vi "DeQ Valve State.vi"(8 "error in (no error)":errorcluster, 11 "Capillary Line in":refnum<class "Capillary Line.lvclass">) -> (0 "error out":errorcluster, 3 "Capillary Line out":refnum<class "Capillary Line.lvclass">)   [LabVIEW 2015, in "cRIO-Carbondioxide.lvlib" / "CO2-Actor.lvlib" / "Capillary Line.lvclass"]
uses:
  Capillary Line.lvclass
  Capillary Line.lvclass/Capillary Line.ctl
panel:
  out "timed out?":bool
  out "State":u16
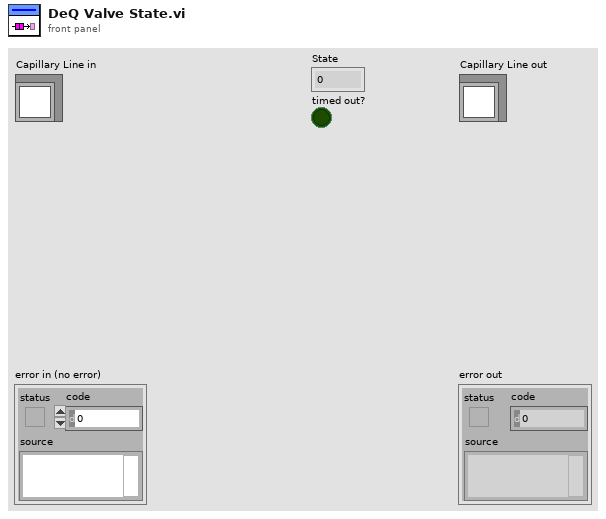
[diagram p1: front panel]
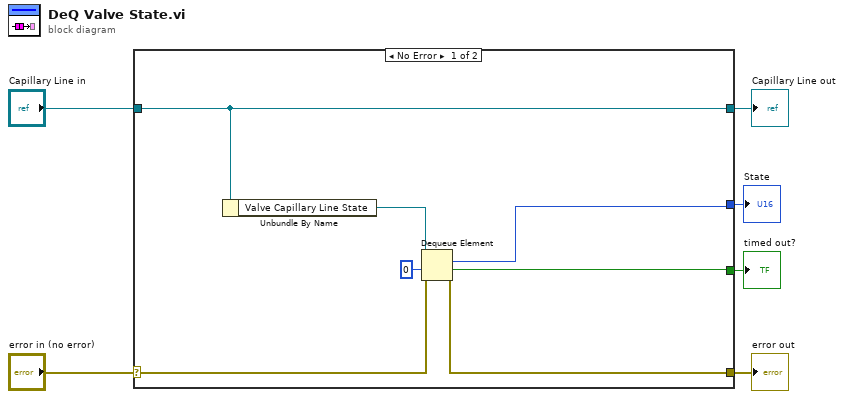
[diagram p0: block diagram]
diagram:
  n1 = case shown="No Error" "error in (no error)" {
    selector: "error in (no error)" -> [w11 w15]
    tunnel: [w10 w15] -> w5
    tunnel: [w13 w14] -> w3
    tunnel: "Capillary Line in" -> [w13 w14]
    tunnel: [w8 _] -> w2
    tunnel: [w7 _] -> w1
    frame No Error {
      n2 = Unbundle By Name(w13) -> ("Valve Capillary Line State"=w12:refnum<queue>)
      n3 = Dequeue Element(queue=w12, timeout in ms (-1)=0, error in (no error)=w11) -> (element=w8:u16, timed out?=w7:bool, error out=w10:errorcluster)  [unwired: 1 out]
    }
    frame Error {
    }
  }
  "error out" <- w5
  "Capillary Line out" <- w3
  "State" <- w2
  "timed out?" <- w1
